vi "Get to lower angle.vi"(0 "Intake Info In":T1, 1 "Kick Info":T2, 2 "error in (no error)":errorcluster) -> (3 "Intake Info Out":T1, 4 "Kick Info":T2, 5 "Finished":bool, 6 "error out":errorcluster)   [LabVIEW 2013]
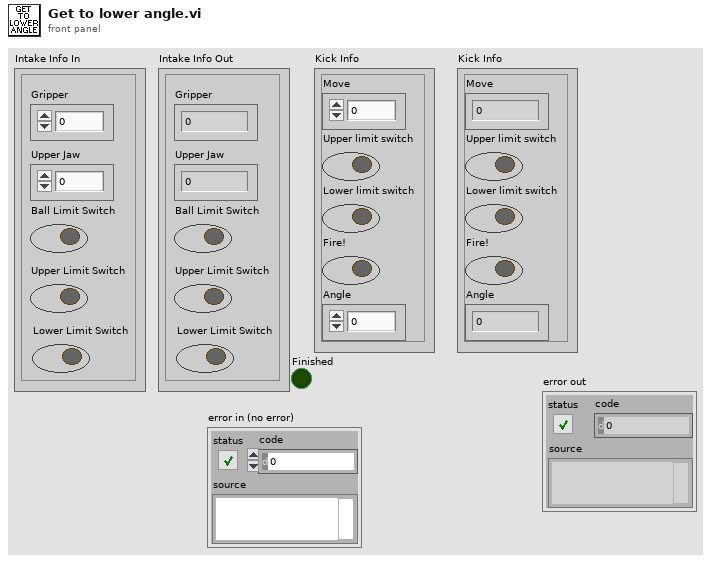
[diagram p1: front panel]
types:
  T1 = cluster{"Gripper":dbl, "Upper Jaw":dbl, "Ball Limit Switch":bool, "Upper Limit Switch":bool, "Lower Limit Switch ":bool}
  T2 = cluster{"Move":dbl, "Upper limit switch":bool, "Lower limit switch ":bool, "Fire!":bool, "Angle":dbl}
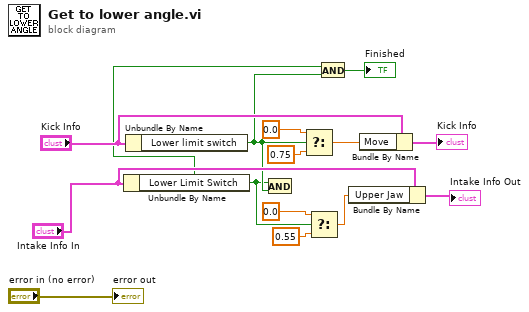
[diagram p0: block diagram]
diagram:
  n1 = Unbundle By Name("Intake Info In") -> ("Lower Limit Switch"=w2:bool)
  n2 = Unbundle By Name("Kick Info") -> ("Lower limit switch"=w3:bool)
  n3 = And(x=w2, y=w3) -> ()  [unwired: 1 out]
  n4 = Select(t=0.0 ("f"), s=w3, f=0.75 ("t")) -> (s? t:f=w10:dbl)
  n5 = Select(t=0.0, s=w2, f=0.55) -> (s? t:f=w6:dbl)
  n6 = And(x=w2, y=w3) -> (x .and. y?=→"Finished":bool)
  n7 = Bundle By Name(cluster="Intake Info In", "Upper Jaw"=w6) -> (→"Intake Info Out":T1)
  n8 = Bundle By Name(cluster="Kick Info", "Move"=w10) -> (→"Kick Info":T2)
  "error out" <- "error in (no error)"
